vi "write_udc_continuous.vi"(1 "Value":dbl, 2 "Hex Address":u16 format="%x", 3 "TCP Connection Refnum in":refnum<k5>) -> ()   [LabVIEW 2011]
uses:
  <vilib>/NI Modbus.llb/MB Ethernet Master Query Write Multiple Registers (poly).vi
panel:
  out "Error Out":errorcluster
  out "Exception Code":u8 format="%.0x"
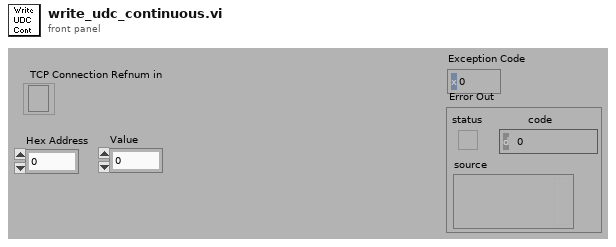
[diagram p1: front panel]
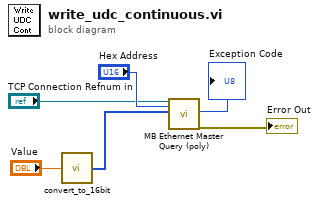
[diagram p0: block diagram]
diagram:
  n1 = call "convert_to_16bit.vi"("Floating point"="Value") -> ("Output Array"=w5:u16[])
  n2 = call-poly <vilib>:"MB Ethernet Master Query (poly).vi"("TCP Connection Refnum in"="TCP Connection Refnum in", "Starting Address"="Hex Address", "Registers"=w5) -> ("Exception Code"=→"Exception Code":u8, "error out"=→"Error Out":errorcluster)  [unwired: 3 in, 12 out]
